vi "例10.5  利用底层函数连续采集图像（设置参数）.vi"() -> ()   [LabVIEW 2017]
doc: "The Grab VI acquires images continuously and displays the images in an image control using low-level acquisition VIs. A grab is appropriate for high-speed applications in which you need to process only one image at a time."
uses:
  <vilib>/userdefined/High Color/IMAQdx.ctl
  <vilib>/vision/driver/IMAQdx.llb/IMAQdx Acquisition Mode.ctl
  <vilib>/vision/driver/IMAQdx.llb/IMAQdx Buffer Number Mode.ctl
  <vilib>/vision/driver/NI_Vision_Acquisition_Software.lvlib
  <resource>/objmgr/imaqdx.rc
panel:
  in  "VideoMode":u32
  in  "Camera Name":T1
  out "Buffer Number":u32
  out "Image":T2(plugin-control)
  in  "stop":bool
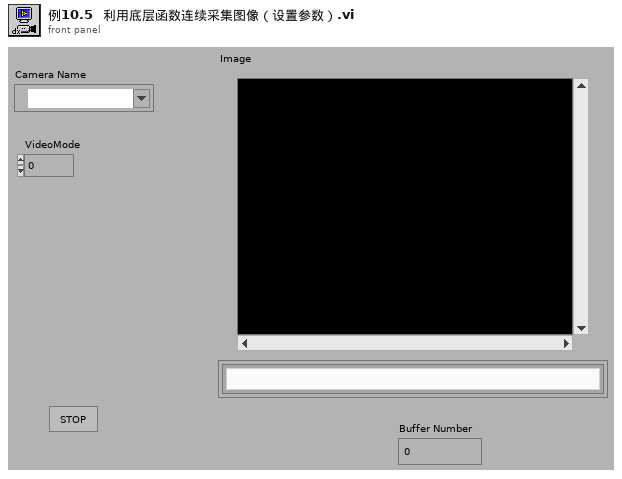
[diagram p1: front panel]
types:
  T1 = typedef "IMAQdx.ctl" = refnum<k21>
  T2 = typedef "IMAQ Image.ctl" = refnum<image>
  T3 = typedef "NI_Vision_Acquisition_Software.lvlib/IMAQdx Acquisition Mode.ctl" = enum32{"One Shot", "Continuous"}
  T4 = typedef "NI_Vision_Acquisition_Software.lvlib/IMAQdx Buffer Number Mode.ctl" = enum32{"Next", "Last", "Buffer Number", "Every", "Last New"}
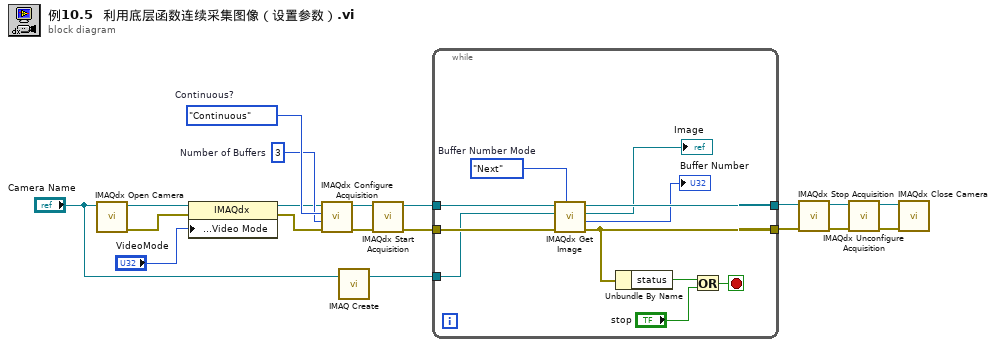
[diagram p0: block diagram]
diagram:
  w12 = u32 3  # Number of Buffers
  w13 = IMAQdx_Acquisition_Mode."Continuous"  # Continuous?
  n1 = call <vilib>:"IMAQdx Open Camera.vi"("Session In"="Camera Name") -> ("error out"=w4:errorcluster, "Session Out"=w5:T1)  [unwired: 2 in, 7 out]
  n2 = property class="IMAQdx"(reference=w5, error in=w4, "Acquisition Attributes:Video Mode"="VideoMode") -> (reference out=w3:T1, error out=w2:errorcluster)
  n3 = call <vilib>:"IMAQdx Configure Acquisition.vi"("error in"=w2, "Number of Buffers"=w12, "Continuous?"=w13, "Session In"=w3) -> ("error out"=w15:errorcluster, "Session Out"=w17:T1)  [unwired: 6 out]
  n4 = call "IMAQ Create"("Image Name"="Camera Name") -> ("New Image"=w19:T2)  [unwired: 3 in, 2 out]
  n5 = call <vilib>:"IMAQdx Start Acquisition.vi"("error in"=w15, "Session In"=w17) -> ("error out"=w14:errorcluster, "Session Out"=w16:T1)  [unwired: 8 out]
  n6 = while {
    tunnel: [w24] -> w10
    tunnel: w14 -> [w26]
    tunnel: w16 -> [w27]
    tunnel: [w23] -> w11
    tunnel: w19 -> [w25]
    stop <- w30 stop-if-true
    w20 = IMAQdx_Buffer_Number_Mode."Next"  # Buffer Number Mode
    n7 = call <vilib>:"IMAQdx Get Image.vi"("Buffer Number Mode (Next)"=w20, "error in"=w26, "Image In"=w25, "Session In"=w27) -> ("error out"=w23:errorcluster, "Buffer Number Out"=→"Buffer Number":u32, "Image Out"=→"Image":T2, "Session Out"=w24:T1)  [unwired: 1 in, 3 out]
    n8 = Unbundle By Name(w23) -> ("status"=w29:bool)
    n9 = Or(x=w29, y="stop") -> (x .or. y?=w30:bool)
  }
  n10 = call <vilib>:"IMAQdx Stop Acquisition.vi"("error in"=w11, "Session In"=w10) -> ("error out"=w6:errorcluster, "Session Out"=w7:T1)  [unwired: 8 out]
  n11 = call <vilib>:"IMAQdx Unconfigure Acquisition.vi"("error in"=w6, "Session In"=w7) -> ("error out"=w9:errorcluster, "Session Out"=w8:T1)  [unwired: 8 out]
  n12 = call <vilib>:"IMAQdx Close Camera.vi"("error in"=w9, "Session In"=w8) -> ()  [unwired: 10 out]
